vi "Message type.vi"(11 "IInternalMessage in":refnum<class "IInternalMessage.lvclass">) -> (2 "Internal message type":T1, 3 "IInternalMessage out":refnum<class "IInternalMessage.lvclass">)   [LabVIEW 2020, in "wamplv.lvlib" / "IInternalMessage.lvclass"]
uses:
  IInternalMessage.lvclass
  TypeDefs/Internal message type.ctl
  wamplv.lvlib
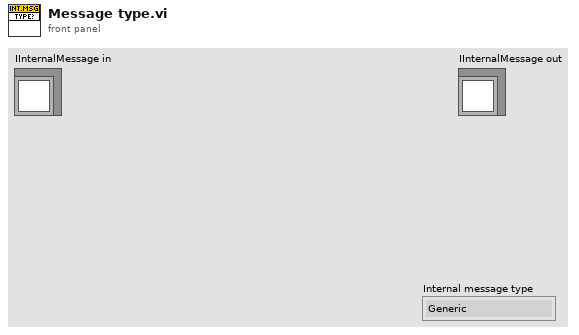
[diagram p1: front panel]
types:
  T1 = typedef "wamplv.lvlib/Internal message type.ctl" = enum16{"Generic", "Generic with write output", "Handle Result", "Handle Error", "Handle Abort", "Handle Welcome", "Handle Goodbye", "Send abort"}
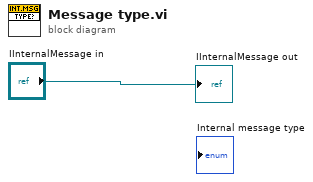
[diagram p0: block diagram]
diagram:
  "IInternalMessage out" <- "IInternalMessage in"
